vi "First Step.vi"(8 "error in (no error)":errorcluster, 11 "Microwave Freq Scan.lvclass in":refnum<class "Microwave Freq Scan.lvclass">) -> (0 "error out":errorcluster, 2 "Current Position":dbl, 3 "Microwave Freq Scan.lvclass out":refnum<class "Microwave Freq Scan.lvclass">)   [LabVIEW 2012, in "Microwave Freq Scan.lvclass"]
doc: "(Dynamic) Reset the instrument and prepare to scan. Goto step #0 - the first step. If desired, the scanner may do this in a different way than usual (i.e. by preparing to move a long distance, or reset to home position.)"
uses:
  Microwave Freq Scan.lvclass
  Scanner/Scanner.lvclass
  Instruments/Utility Classes/Scannable/Scannable.lvclass
  Instruments/Microwave/Agilent PSG MXG Series/Agilent PSG MXG Series.lvlib
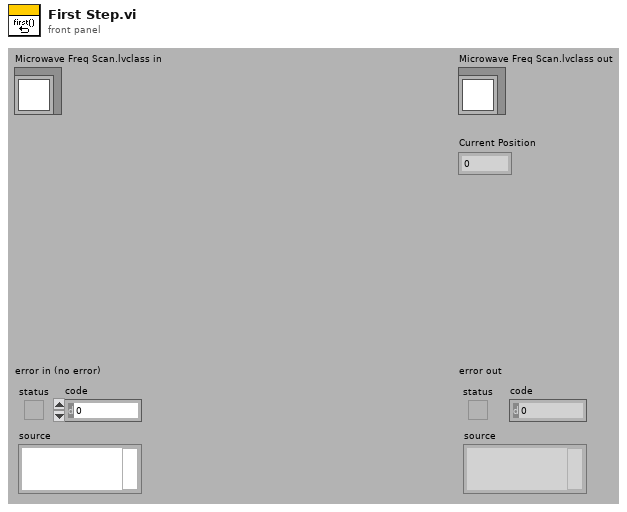
[diagram p1: front panel]
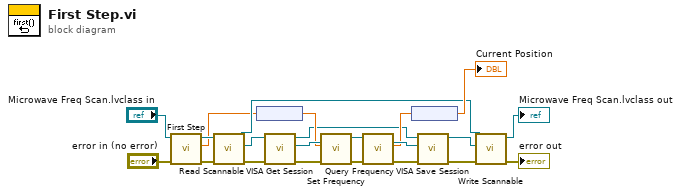
[diagram p0: block diagram]
diagram:
  n1 = call-parent "First Step.vi"("error in (no error)"="error in (no error)", "Scanner.lvclass in"="Microwave Freq Scan.lvclass in") -> ("error out"=w14:errorcluster, "Current Position"=w1:dbl, "Scanner.lvclass out"=w20:refnum<class "Microwave Freq Scan.lvclass">)  [unwired: 7 out]
  n2 = call-dynamic "Read Scannable.vi"("error in (no error)"=w14, "Scanner.lvclass in"=w20) -> ("error out"=w15:errorcluster, "Scannable.lvclass"=w19:refnum<class "Scannable.lvclass">, "Scanner.lvclass out"=w6:refnum<class "Microwave Freq Scan.lvclass">)  [unwired: 7 out]
  n3 = node(w1) -> (w17:dbl[unit])
  n4 = call-dynamic "VISA Get Session.vi"("error in (no error)"=w15, "Instrument.lvclass in"=w19) -> ("error out"=w16:errorcluster, "VISA Resource Name"=w18:refnum<visa-resource-name>, "Instrument.lvclass out"=w7:refnum<class "Scannable.lvclass">)  [unwired: 7 out]
  n5 = call "Set Frequency.vi"("error in (no error)"=w16, "Frequency"=w17, "VISA resource name"=w18) -> ("error out"=w12:errorcluster, "VISA resource name out"=w13:refnum<visa-resource-name>)  [unwired: 7 out]
  n6 = call "Query Frequency.vi"("error in (no error)"=w12, "VISA resource name"=w13) -> ("error out"=w10:errorcluster, "Frequency"=w9:dbl[unit], "VISA resource name out"=w11:refnum<visa-resource-name>)  [unwired: 7 out]
  n7 = node(w9) -> (→"Current Position":dbl)
  n8 = call-dynamic "VISA Save Session.vi"("error in (no error)"=w10, "VISA Resource Name"=w11, "Instrument.lvclass in"=w7) -> ("error out"=w3:errorcluster, "Instrument.lvclass out"=w4:refnum<class "Scannable.lvclass">)  [unwired: 7 out]
  n9 = call-dynamic "Write Scannable.vi"("error in (no error)"=w3, "Scannable.lvclass"=w4, "Scanner.lvclass in"=w6) -> ("error out"=→"error out":errorcluster, "Scanner.lvclass out"=→"Microwave Freq Scan.lvclass out":refnum<class "Microwave Freq Scan.lvclass">)  [unwired: 7 out]
